vi "Encode Text Payload.vi"(8 "error in (no error)":errorcluster, 11 "Text":string) -> (0 "error out":errorcluster, 3 "Packet":string)   [LabVIEW 2023, in "WebSocket.lvclass"]
uses:
  WebSocket.lvclass
  private/Fixed Header.ctl
  private/OpCode.ctl
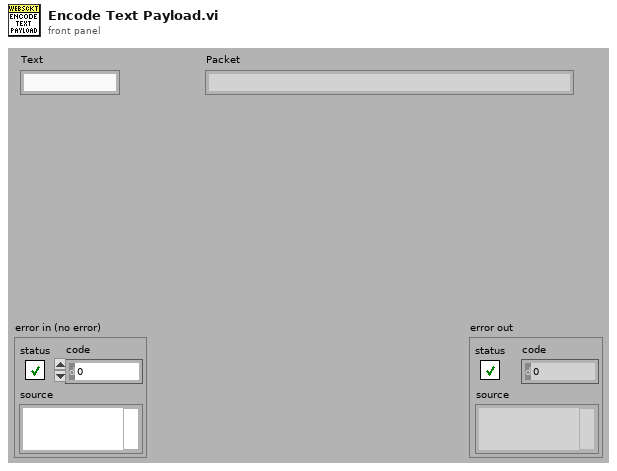
[diagram p1: front panel]
types:
  T1 = typedef "WebSocket.lvclass/Fixed Header.ctl" = cluster{"FIN":bool, "RSVD1":bool, "RSVD2":bool, "RSVD3":bool, "OpCode":T2, "MASK":bool, "Len":u8}
  T2 = typedef "WebSocket.lvclass/OpCode.ctl" = enum16{"Cont.", "Text", "Binary", "NonCtl3", "NonCtl4", "NonCtl5", "NonCtl6", "NonCtl7", "Close", "Ping", "Pong", "Rsvd11", "Rsvd12", "Rsvd13", "Rsvd14", "Rsvd15"}
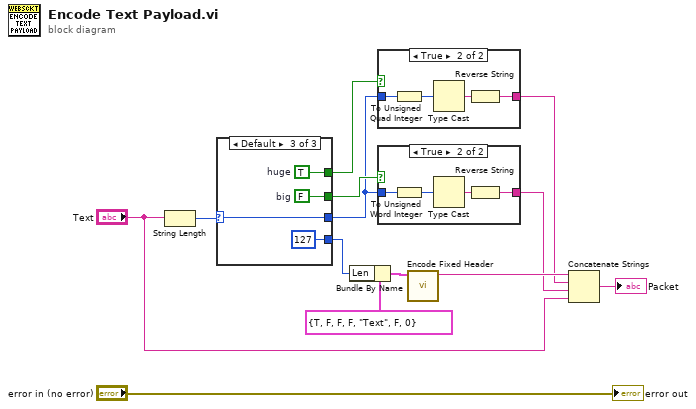
[diagram p0: block diagram]
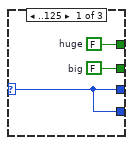
[diagram p4: hidden frame]
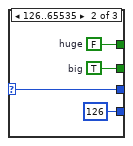
[diagram p5: hidden frame]
diagram:
  n1 = String Length(string="Text") -> (length=w12:i32)
  n2 = case shown="Default" w12 {
    selector: w12 -> [w14 w20 w24]
    tunnel: [w14 w20 w24] -> w6
    tunnel: [w16 w19 w23] -> w7
    tunnel: [w15 w18 w22] -> w8
    tunnel: [w14 126 ("Len") 127 ("Len")] -> w9
    frame ..125 {
      w16 = FALSE  # big
      w15 = FALSE  # huge
    }
    frame 126..65535 {
      w19 = TRUE  # big
      w18 = FALSE  # huge
    }
    frame Default {
      w23 = FALSE  # big
      w22 = TRUE  # huge
    }
  }
  n3 = Bundle By Name(cluster=T1 {"FIN"=TRUE, "RSVD1"=FALSE, "RSVD2"=FALSE, "RSVD3"=FALSE, "OpCode"=enum."Text", "MASK"=FALSE, "Len"=0} ("Fixed Header"), "Len"=w9) -> (w10:T1)
  n4 = case shown="True" w8 {
    tunnel: w6 -> [_ w28]
    tunnel: [_ w25] -> w4
    frame False {
    }
    frame True {
      n5 = To Unsigned Quad Integer(1:w28) -> (0:w27:u64)
      n6 = Type Cast(x=w27) -> (*(type *) &x=w26:string)  [unwired: 1 in]
      n7 = Reverse String(1:w26) -> (0:w25:string)
    }
  }
  n8 = case shown="True" w7 {
    tunnel: w6 -> [_ w32]
    tunnel: [_ w29] -> w3
    frame False {
    }
    frame True {
      n9 = To Unsigned Word Integer(number=w32) -> (unsigned 16bit integer=w31:u16)
      n10 = Type Cast(x=w31) -> (*(type *) &x=w30:string)  [unwired: 1 in]
      n11 = Reverse String(1:w30) -> (0:w29:string)
    }
  }
  n12 = call "Encode Fixed Header.vi"("Fixed Header"=w10) -> ("String"=w5:string)  [unwired: 9 in, 1 out]
  n13 = Concatenate Strings(w5, w4, w3, "Text") -> (→"Packet":string)
  "error out" <- "error in (no error)"
